vi "FYP_VI_MIDI_Open.vi"(7 "deviceID":u32) -> (0 "midiOutOpen Error Code":i32, 3 "midiOut":i32)   [LabVIEW 2013]
uses:
  winmm.dll
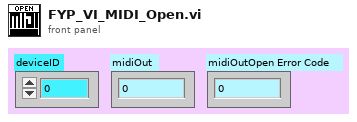
[diagram p1: front panel]
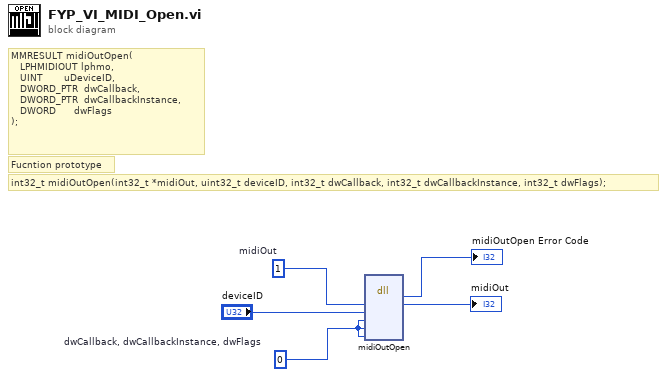
[diagram p0: block diagram]
diagram:
  w3 = 0  # dwCallback, dwCallbackInstance, dwFlags
  w5 = 1  # midiOut
  # "Fucntion prototype"
  # "int32_t midiOutOpen(int32_t *midiOut, uint32_t deviceID, int32_t dwCallback, int32_t dwCallbackInstance, int32_t dwFlags);"
  # "MMRESULT midiOutOpen(\n   LPHMIDIOUT lphmo,\n   UINT       uDeviceID,\n   DWORD_PTR  dwCallback,\n   DWORD_PTR  dwCallbackInstance,\n   DWORD      dwFlags\n);"
  n1 = dll-call lib="winmm.dll" fn="midiOutOpen"("midiOut"=w5, "deviceID"="deviceID", "dwCallback"=w3, "dwCallbackInstance"=w3, "dwFlags"=w3) -> ("return type"=→"midiOutOpen Error Code":i32, "midiOut"=→"midiOut":i32)  [unwired: 7 in, 2 out]
